vi "Fit Data.vi"(8 "error in":errorcluster, 10 "Data In":dbl[](array[numeric]), 11 "LRS in":refnum<class "LRS.lvclass">) -> (0 "error out":errorcluster, 3 "LRS out":refnum<class "LRS.lvclass">)   [LabVIEW 2014, in "Exponential Fit Library.lvlib" / "LRS.lvclass"]
doc: "LRS is the retangular integration solution of linear least squares, this techniques solves the following linear system \n\n| N SI St | |a0 | | Sf |\n| SI SII StI | | a1| = |SfI |\n| St StI Stt | | a2 | |Sft |\n\nwhere N is the numberr of points in the exponential and Sx represents the sum of term x and Sxy represents the sum of the product of two terms at each point evaluated. I is the running integral of the signal x (evaluated using rectangular integration, or sum(f_i*t_i) where f is the value of the exponential at point i and t is the time at point i (in this case, dt is = 1). The matrix A is positive definite (apparent from the structure above) and we can use Cholesky decomposition to solve for the vector a. We can then evaluate tau using this vector:\n\nbeta = ln(1-a1)\n\nand \n\ntau = dt/beta"
uses:
  LRS.lvclass
  <vilib>/Analysis/baseanly.llb/Matrix Type of Inverse Matrix.ctl
  Fit Exponential.lvclass/Fit Exponential.ctl
  LRS.lvclass/LRS.ctl
  <vilib>/Analysis/7linalg.llb/Solve Linear Equations (single right hand).vi
  Read Size.vi
  Read Stt.vi
  Read Ramp.vi
  Read St.vi
  Read Dt.vi
  Write Output.vi
  <vilib>/Analysis/baseanly.llb/Solve Linear Equations By Cholesky.vi
  <vilib>/Analysis/baseanly.llb/Real Matrix to Compact Array.vi
  <vilib>/Analysis/baseanly.llb/Real Compact Tri-Matrix Linear Eqs.vi
  <vilib>/Analysis/Matrix/Numeric/Conversions/Array To Matrix - RA2.vi
  <vilib>/Analysis/7linalg.llb/Solve Linear Eqs (General).vi
  <vilib>/Analysis/7linalg.llb/Solve Linear Eqs (Gen, single right hand).vi
  Fit Exponential.lvclass
  <vilib>/Analysis/NI_AALBase.lvlib
  <vilib>/Analysis/NI_AALPro.lvlib
  <vilib>/Analysis/Matrix/NI_Matrix.lvlib
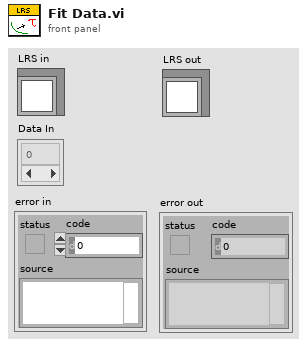
[diagram p1: front panel]
types:
  T1 = cluster{"A":dbl, "B":dbl, "tau":dbl, "e_tau":dbl}
  T2 = typedef "NI_AALBase.lvlib/Matrix Type of Inverse Matrix.ctl" = enum32{"General", "Positive Definite", "Lower Triangular", "Upper Triangular"}
  T3 = typedef "NI_Matrix.lvlib/RealMatrix.ctl" = dbl[][]
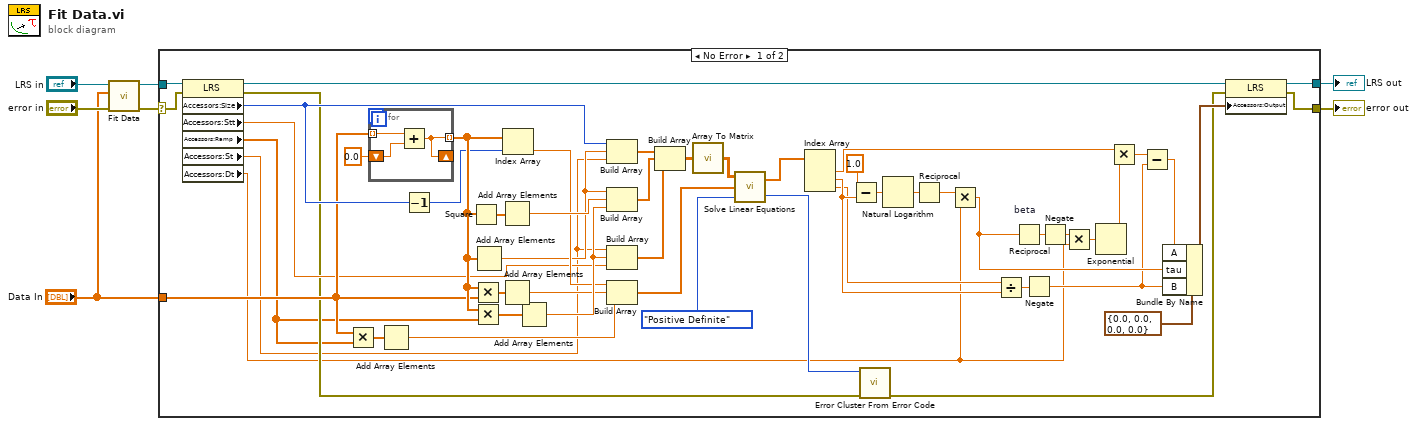
[diagram p0: block diagram]
diagram:
  n1 = call-parent "Fit Data.vi"("error in"="error in", "Data In"="Data In", "Fit Exponential in"="LRS in") -> ("error out"=w5:errorcluster, "Fit Exponential out"=w4:refnum<class "LRS.lvclass">)  [unwired: 7 in]
  n2 = case shown="No Error" w5 {
    selector: w5 -> [w31 w64]
    tunnel: w4 -> [w35 w65]
    tunnel: "Data In" -> [w33 _]
    tunnel: [w16 w65] -> w2
    tunnel: [w9 w64] -> w1
    frame No Error {
      n3 = property class="LRS"(reference=w35, error in=w31) -> (reference out=w17:refnum<class "LRS.lvclass">, error out=w30:errorcluster, "Accessors:Size"=w34:i32, "Accessors:Stt"=w32:dbl, "Accessors:Ramp"=w27:dbl[], "Accessors:St"=w28:dbl, "Accessors:Dt"=w8:dbl)
      n4 = Multiply(x=w33, y=w27) -> (x*y=w52:dbl[])
      n5 = for {
        tunnel: w33 -> [w63] mode=indexing
        tunnel: [w61] -> w41 mode=indexing
        shift-right: [w61] -> _
        shift-left: 0.0 -> [w62]
        n6 = Add(x=w63, y=w62) -> (x+y=w61:dbl)
      }
      n7 = Add Array Elements ("Sft")(numeric array=w52) -> (sum=w51:dbl)
      n8 = Decrement(x=w34) -> (x-1=w40:i32)
      n9 = Square(x=w41) -> (x^2=w59:dbl[])
      n10 = Multiply(x=w41, y=w33) -> (x*y=w58:dbl[])
      n11 = Multiply(x=w41, y=w27) -> (x*y=w57:dbl[])
      n12 = Add Array Elements ("SI")(numeric array=w41) -> (sum=w39:dbl)
      n13 = Add Array Elements ("SII")(numeric array=w59) -> (sum=w56:dbl)
      n14 = Add Array Elements ("SfI")(numeric array=w58) -> (sum=w53:dbl)
      n15 = Index Array(array=w41, index=w40) -> (element=w54:dbl)
      n16 = Add Array Elements ("StI")(numeric array=w57) -> (sum=w55:dbl)
      n17 = Build Array(w34, w39, w28) -> (w49:dbl[])
      n18 = Build Array(w39, w56, w55) -> (w48:dbl[])
      n19 = Build Array(w28, w55, w32) -> (w47:dbl[])
      n20 = Build Array(w54, w53, w51) -> (w50:dbl[])
      n21 = Build Array(w49, w48, w47) -> (w46:dbl[][])
      n22 = call-poly <vilib>:"Array To Matrix.vi"("Real 2D Array"=w46) -> ("Real Matrix"=w45:T3)
      n23 = call-poly <vilib>:"Solve Linear Equations.vi"("matrix type"=Matrix_Type_of_Inverse_Matrix."Positive Definite", "Known Vector"=w50, "Input Matrix"=w45) -> ("error"=w36:i32, "Solution Vector"=w29:dbl[])
      n24 = Index Array(array=w29) -> (element #1=w21:dbl, element #2=w19:dbl, element #3=w18:dbl)  [unwired: 3 in]
      n25 = Subtract(x=1.0, y=w19) -> (x-y=w43:dbl)
      n26 = call <vilib>:"Error Cluster From Error Code.vi"("error in (no error)"=w30, "error code (0)"=w36) -> ("error out"=w10:errorcluster)  [unwired: 7 in]
      n27 = Natural Logarithm(1:w43) -> (0:w42:dbl)
      n28 = Reciprocal(x=w42) -> (1/x=w38:dbl)
      n29 = Multiply(x=w38, y=w8) -> (x*y=w13:dbl)
      n30 = Divide(x=w18, y=w19) -> (x/y=w20:dbl)
      n31 = Reciprocal "beta"(x=w13) -> (1/x=w26:dbl)
      n32 = Negate(x=w20) -> (-x=w12:dbl)
      n33 = Negate(x=w26) -> (-x=w25:dbl)
      n34 = Multiply(x=w25, y=w8) -> (x*y=w24:dbl)
      n35 = Exponential(1:w24) -> (0:w22:dbl)
      n36 = Multiply(x=w21, y=w22) -> (x*y=w23:dbl)
      n37 = Subtract(x=w23, y=w12) -> (x-y=w14:dbl)
      n38 = Bundle By Name(cluster=T1 {"A"=0.0, "B"=0.0, "tau"=0.0, "e_tau"=0.0} ("Output"), "A"=w14, "tau"=w13, "B"=w12) -> (w11:T1)
      n39 = property class="LRS"(reference=w17, error in=w10, "Accessors:Output"=w11) -> (reference out=w16:refnum<class "LRS.lvclass">, error out=w9:errorcluster)
    }
    frame Error {
    }
  }
  "error out" <- w1
  "LRS out" <- w2
